vi "XY2Heading.vi"(8 "X":dbl format="%#_13g", 11 "Y":dbl format="%#_13g") -> (2 "heading":dbl)   [LabVIEW 2016]
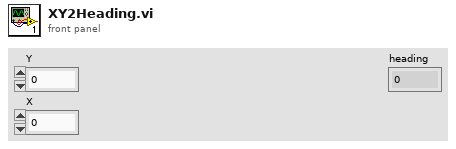
[diagram p1: front panel]
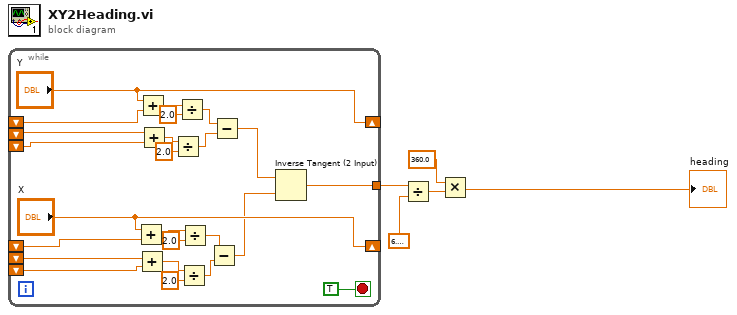
[diagram p0: block diagram]
diagram:
  n1 = while {
    shift-right: ["Y"] -> _
    shift-left: _ -> [w23]
    shift-right: ["X"] -> _
    shift-left: _ -> [w28]
    shift-left: _ -> [w22]
    shift-left: _ -> [w21]
    shift-left: _ -> [w26]
    shift-left: _ -> [w25]
    tunnel: [w8] -> w5
    stop <- TRUE stop-if-true
    n2 = Add(x="X", y=w28) -> (x+y=w14:dbl)
    n3 = Add(x=w26, y=w25) -> (x+y=w15:dbl)
    n4 = Add(x="Y", y=w23) -> (x+y=w20:dbl)
    n5 = Add(x=w22, y=w21) -> (x+y=w13:dbl)
    n6 = Divide(x=w13, y=2.0) -> (x/y=w9:dbl)
    n7 = Divide(x=w20, y=2.0) -> (x/y=w12:dbl)
    n8 = Divide(x=w15, y=2.0) -> (x/y=w10:dbl)
    n9 = Divide(x=w14, y=2.0) -> (x/y=w11:dbl)
    n10 = Subtract(x=w11, y=w10) -> (x-y=w6:dbl)
    n11 = Subtract(x=w12, y=w9) -> (x-y=w7:dbl)
    n12 = Inverse Tangent (2 Input)(1:w6, 2:w7) -> (0:w8:dbl)
  }
  n13 = Divide(x=w5, y=6.283185307179586) -> (x/y=w3:dbl)
  n14 = Multiply(x=360.0, y=w3) -> (x*y=→"heading":dbl)
